vi "步响应t2.vi"(0 "X_Peaks":dbl[](array[numeric]), 1 "Y_Peaks":dbl[](array[numeric]), 2 "h0":dbl, 3 "X_valleys":dbl[](array[numeric]), 4 "Y_valleys":dbl[](array[numeric])) -> (5 "t2":dbl)   [LabVIEW 2013]
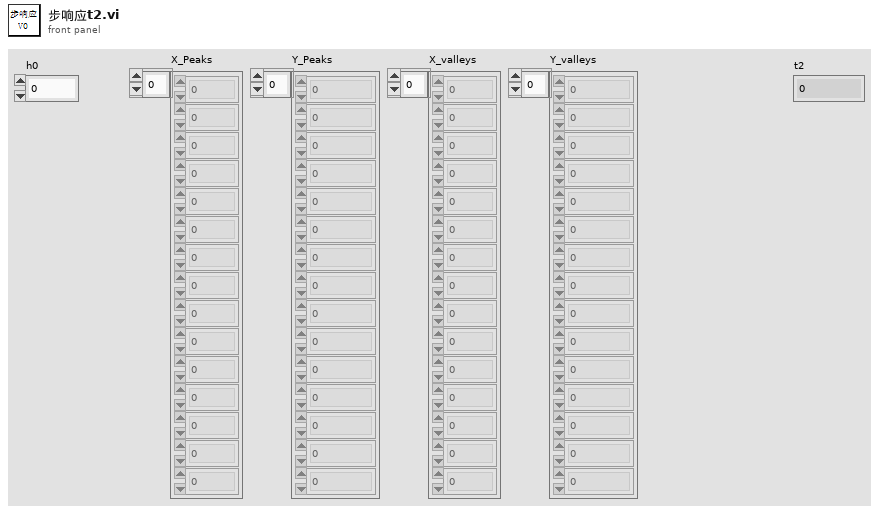
[diagram p1: front panel]
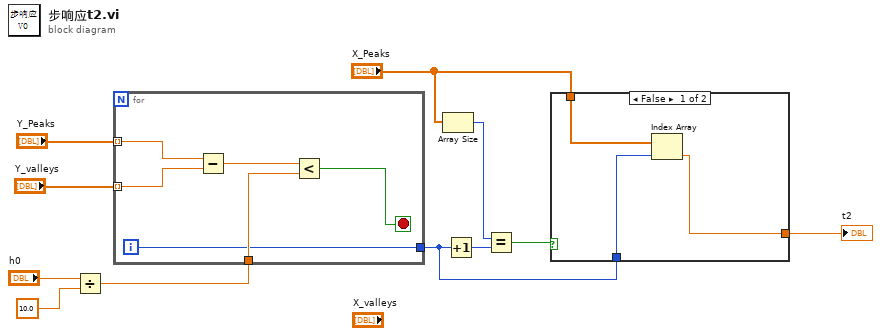
[diagram p0: block diagram]
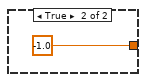
[diagram p2: hidden frame]
diagram:
  n1 = Divide(x="h0", y=10.0) -> (x/y=w7:dbl)
  n2 = for {
    tunnel: "Y_Peaks" -> [w17] mode=indexing
    tunnel: "Y_valleys" -> [w16] mode=indexing
    tunnel: w7 -> [w14]
    tunnel: [w12] -> w1
    i -> [w12]
    stop <- w13 stop-if-true
    n3 = Subtract(x=w17, y=w16) -> (x-y=w15:dbl)
    n4 = Less?(x=w15, y=w14) -> (x < y?=w13:bool)
  }
  n5 = Array Size(array="X_Peaks") -> (size(s)=w6:i32)
  n6 = Increment(x=w1) -> (x+1=w2:i32)
  n7 = Equal?(x=w6, y=w2) -> (x = y?=w5:bool)
  n8 = case shown="False" w5 {
    tunnel: [w18 -1.0] -> w4
    tunnel: "X_Peaks" -> [w20 _]
    tunnel: w1 -> [w19 _]
    frame False {
      n9 = Index Array(array=w20, index=w19) -> (element=w18:dbl)
    }
    frame True {
    }
  }
  "t2" <- w4
